vi "Left Motor Test.vi"   [LabVIEW 2015]
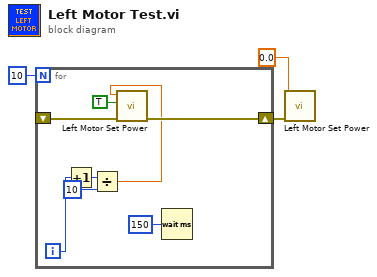
[diagram p0: block diagram]
diagram:
  n1 = for {
    N: 10 -> [_]
    shift-right: [w11] -> w2
    shift-left: _ -> [w10]
    i -> [w8]
    n2 = Increment(x=w8) -> (x+1=w7:i32)
    n3 = Divide(x=w7, y=10) -> (x/y=w5:dbl)
    n4 = call "Left Motor Set Power.vi"("error in"=w10, "Disable Ramp"=TRUE, "Output"=w5) -> ("error out"=w11:errorcluster)  [unwired: 8 in]
    n5 = Wait (ms)(milliseconds to wait=u32 150) -> ()  [unwired: 1 out]
  }
  n6 = call "Left Motor Set Power.vi"("error in"=w2, "Output"=0.0) -> ()  [unwired: 9 in, 1 out]
